vi "Search Both Address.vi"(1 "Address U":string[](array[string]), 2 "Address C":string[](array[string]), 3 "Key":string[](array[string]), 10 "sorted array":string[](array[string])) -> (5 "Found Key   2":string, 6 "Found Address  2":string, 8 "Match!  2":bool)   [LabVIEW 2020]
uses:
  fc8f06de-4352-3fe5-ca1e-410684fae83f.vi
  c43f61cc-456e-3fd0-4807-e93e1587c13f.vi
  fc8f06de-4352-3fe5-ca1e-410684fae83f.vi/d4db2432-cc9c-482c-8957-dac855435ef6.vi
  fc8f06de-4352-3fe5-ca1e-410684fae83f.vi/86fbf154-bd7b-49a2-8ab2-a837b2a95f24.vi
  fc8f06de-4352-3fe5-ca1e-410684fae83f.vi/3b95b01e-1ec2-4565-bcd9-7606a5281010.vi
  fc8f06de-4352-3fe5-ca1e-410684fae83f.vi/96a08935-737a-44b2-979c-a81d56408f7e.vi
  c43f61cc-456e-3fd0-4807-e93e1587c13f.vi/d4db2432-cc9c-482c-8957-dac855435ef6.vi
  c43f61cc-456e-3fd0-4807-e93e1587c13f.vi/86fbf154-bd7b-49a2-8ab2-a837b2a95f24.vi
  c43f61cc-456e-3fd0-4807-e93e1587c13f.vi/3b95b01e-1ec2-4565-bcd9-7606a5281010.vi
  c43f61cc-456e-3fd0-4807-e93e1587c13f.vi/96a08935-737a-44b2-979c-a81d56408f7e.vi
  fc8f06de-4352-3fe5-ca1e-410684fae83f.vi/d4db2432-cc9c-482c-8957-dac855435ef6.vi/6eaecd13-6e48-4772-a921-b51ebdf84d88.vi
  fc8f06de-4352-3fe5-ca1e-410684fae83f.vi/d4db2432-cc9c-482c-8957-dac855435ef6.vi/d2d5f2b7-06f4-47f6-971c-049c3fdbb653.vi
  fc8f06de-4352-3fe5-ca1e-410684fae83f.vi/3b95b01e-1ec2-4565-bcd9-7606a5281010.vi/6eaecd13-6e48-4772-a921-b51ebdf84d88.vi
  fc8f06de-4352-3fe5-ca1e-410684fae83f.vi/3b95b01e-1ec2-4565-bcd9-7606a5281010.vi/d2d5f2b7-06f4-47f6-971c-049c3fdbb653.vi
  fc8f06de-4352-3fe5-ca1e-410684fae83f.vi/96a08935-737a-44b2-979c-a81d56408f7e.vi/6eaecd13-6e48-4772-a921-b51ebdf84d88.vi
  fc8f06de-4352-3fe5-ca1e-410684fae83f.vi/96a08935-737a-44b2-979c-a81d56408f7e.vi/d2d5f2b7-06f4-47f6-971c-049c3fdbb653.vi
  c43f61cc-456e-3fd0-4807-e93e1587c13f.vi/d4db2432-cc9c-482c-8957-dac855435ef6.vi/6eaecd13-6e48-4772-a921-b51ebdf84d88.vi
  c43f61cc-456e-3fd0-4807-e93e1587c13f.vi/d4db2432-cc9c-482c-8957-dac855435ef6.vi/d2d5f2b7-06f4-47f6-971c-049c3fdbb653.vi
  c43f61cc-456e-3fd0-4807-e93e1587c13f.vi/3b95b01e-1ec2-4565-bcd9-7606a5281010.vi/6eaecd13-6e48-4772-a921-b51ebdf84d88.vi
  c43f61cc-456e-3fd0-4807-e93e1587c13f.vi/3b95b01e-1ec2-4565-bcd9-7606a5281010.vi/d2d5f2b7-06f4-47f6-971c-049c3fdbb653.vi
  c43f61cc-456e-3fd0-4807-e93e1587c13f.vi/96a08935-737a-44b2-979c-a81d56408f7e.vi/6eaecd13-6e48-4772-a921-b51ebdf84d88.vi
  c43f61cc-456e-3fd0-4807-e93e1587c13f.vi/96a08935-737a-44b2-979c-a81d56408f7e.vi/d2d5f2b7-06f4-47f6-971c-049c3fdbb653.vi
  <vilib>/Comparison/Less/Less Functor/Less Functor.lvclass
panel:
  out "Found Key   3":string
  out "Match! 3":bool
  in  "Text Enable 2":bool
  out "Path 3":path
  in  "Text Enable":bool
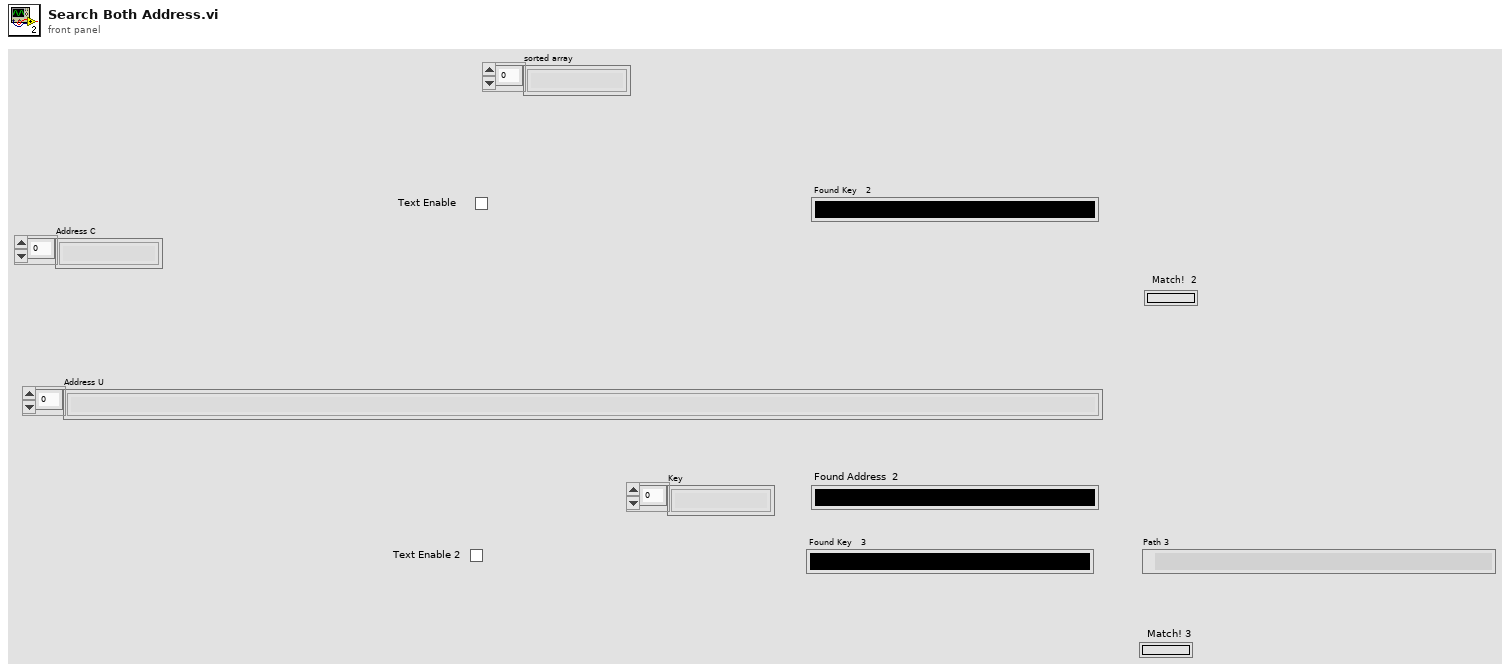
[diagram p1: front panel]
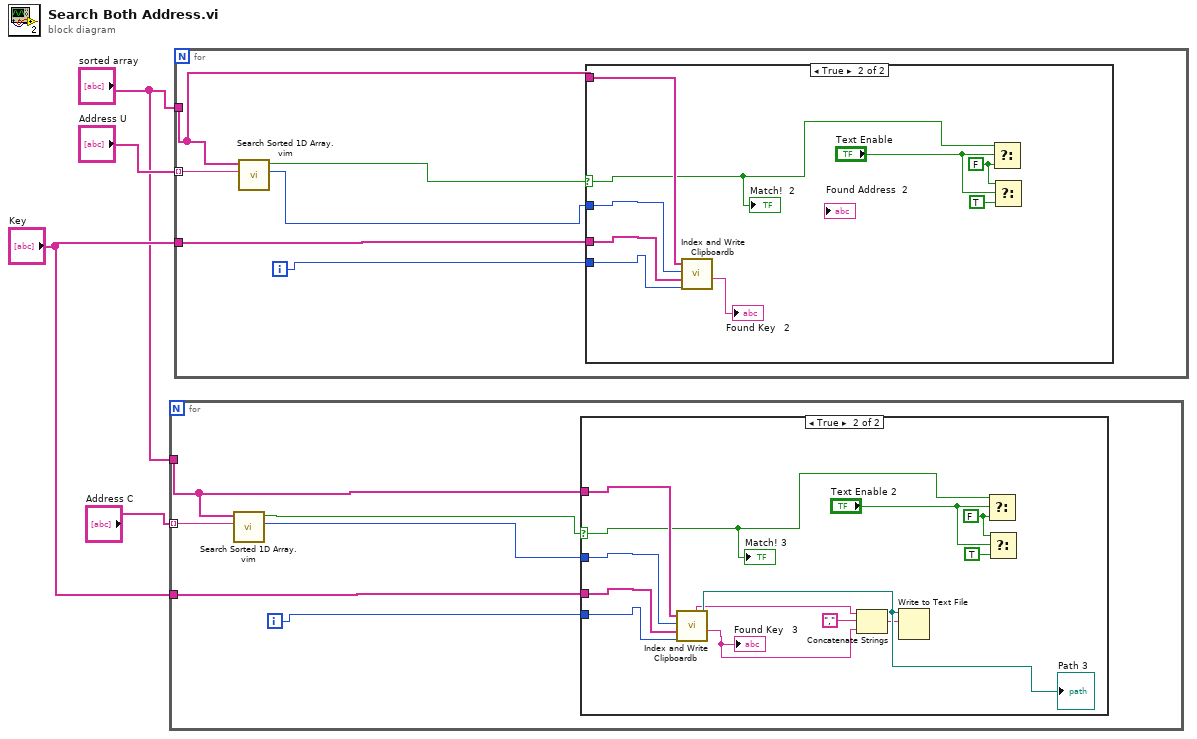
[diagram p0: block diagram]
diagram:
  n1 = for {
    tunnel: "Address C" -> [w9] mode=indexing
    tunnel: "sorted array" -> [w7]
    tunnel: "Key" -> [w10]
    i -> [w8]
    n2 = call "Search Sorted 1D Array.vim"("element"=w9, "sorted 1D array"=w7) -> ("nearest index"=w5:i32, "found?"=w6:bool)  [unwired: 8 in]
    n3 = case shown="True" w6 {
      selector: w6 -> [_ w13]
      tunnel: w7 -> [_ w23]
      tunnel: w5 -> [_ w22]
      tunnel: w10 -> [_ w21]
      tunnel: w8 -> [_ w20]
      frame False {
      }
      frame True {
        w15 = FALSE ("f")
        n4 = call "Index and Write Clipboardb.vi"("Numeric"=w20, "Key Array Out"=w21, "nearest index"=w22, "sorted array"=w23) -> ("Key"=w12:string, "Path"=w19:path, "Address"=w11:string)  [unwired: 5 in]
        "Found Key   3" <- w12
        "Path 3" <- w19
        n5 = Concatenate Strings(w11, "," ("string"), w12) -> (w17:string)
        n6 = Write to Text File(file (use dialog)=w19, text=w17) -> ()  [unwired: 2 in, 3 out]
        n7 = Select(t=w13, s="Text Enable 2", f=w15) -> ()  [unwired: 1 out]
        n8 = Select(t=w15, s="Text Enable 2", f=TRUE) -> ()  [unwired: 1 out]
        "Match! 3" <- w13
      }
    }
  }
  n9 = for {
    tunnel: "Address U" -> [w28] mode=indexing
    tunnel: "sorted array" -> [w24]
    tunnel: "Key" -> [w29]
    i -> [w27]
    n10 = call "Search Sorted 1D Array.vim"("element"=w28, "sorted 1D array"=w24) -> ("nearest index"=w25:i32, "found?"=w26:bool)  [unwired: 8 in]
    n11 = case shown="True" w26 {
      selector: w26 -> [_ w31]
      tunnel: w24 -> [_ w38]
      tunnel: w25 -> [_ w37]
      tunnel: w29 -> [_ w36]
      tunnel: w27 -> [_ w35]
      frame False {
      }
      frame True {
        w32 = FALSE ("f")
        n12 = call "Index and Write Clipboardb.vi"("Numeric"=w35, "Key Array Out"=w36, "nearest index"=w37, "sorted array"=w38) -> ("Key"=→"Found Key   2":string)  [unwired: 5 in, 2 out]
        n13 = Select(t=w31, s="Text Enable", f=w32) -> ()  [unwired: 1 out]
        n14 = Select(t=w32, s="Text Enable", f=TRUE) -> ()  [unwired: 1 out]
        "Match!  2" <- w31
      }
    }
  }
